vi "IsControllerBusy.vi"(0 "System no.":i32, 5 "error in (no error)":errorcluster) -> (14 "Controller Busy":bool, 19 "error out":errorcluster)   [LabVIEW 2026]
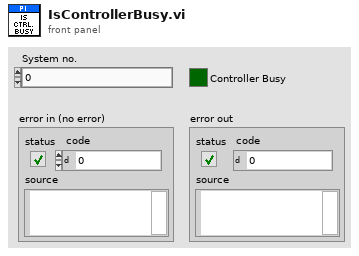
[diagram p1: front panel]
types:
  T1 = typedef "Syntax.ctl" = enum16{"GCS 1.0", "GCS 2.0", "GCS 3.0"}
  T2 = typedef "Status.ctl" = cluster{"Element":string, "Status bits":bool[]}
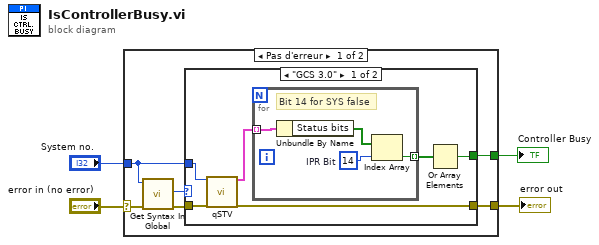
[diagram p0: block diagram]
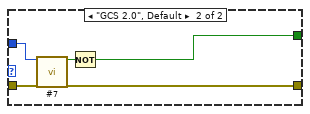
[diagram p2: hidden frame]
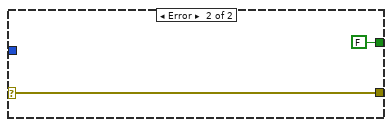
[diagram p3: hidden frame]
diagram:
  n1 = case shown="Pas d'erreur" "error in (no error)" {
    selector: "error in (no error)" -> [w6 w26]
    tunnel: [w10 FALSE] -> w4
    tunnel: [w9 w26] -> w3
    tunnel: "System no." -> [w7 _]
    frame No Error {
      n2 = call "Get Syntax In Global.vi"("error in"=w6, "System no."=w7) -> ("error out"=w5:errorcluster, "Syntax"=w8:T1)  [unwired: 8 in]
      n3 = case shown="\"GCS 3.0\"" w8 {
        tunnel: w7 -> [w16 w25]
        tunnel: w5 -> [w15 w24]
        tunnel: [w14 w23] -> w9
        tunnel: [w12 w21] -> w10
        frame "GCS 3.0" {
          n4 = call "qSTV.vi"("System no."=w16, "error in"=w15) -> ("Status Array"=w13:T2[], "error out"=w14:errorcluster)  [unwired: 16 in]
          n5 = for {
            tunnel: w13 -> [w20] mode=indexing
            tunnel: [w17] -> w11 mode=indexing
            w18 = 14  # IPR Bit
            # "Bit 14 for SYS false"
            n6 = Unbundle By Name(w20) -> ("Status bits"=w19:bool[])
            n7 = Index Array(array=w19, index=w18) -> (element=w17:bool)
          }
          n8 = Or Array Elements(Boolean array=w11) -> (logical OR=w12:bool)
        }
        frame "GCS 2.0", Default {
          n9 = call "#7.vi"("System no."=w25, "error in"=w24) -> ("Ready?"=w22:bool, "error out"=w23:errorcluster)  [unwired: 16 out]
          n10 = Not(x=w22) -> (.not. x?=w21:bool)
        }
      }
    }
    frame Error {
    }
  }
  "Controller Busy" <- w4
  "error out" <- w3
